vi "Get next JSON Value.vi"() -> (1 "Offset past match":i32, 2 "Value start":i32)   [LabVIEW 2013, in "JSON2.lvlib"]
uses:
  JSON2.lvlib
  JSON Value Search.ctl
panel:
  in  "<JSON> Stream 2":string="[\"string\",\"test2\",\"string\",\"t3\",\"string\", \"string\"]"
  out "Time":dbl format="%#_3p"
  in  "index in":i32
  out "Match":string
  out "Enum":T1=enum."Undefined"
  out "Past Match":string
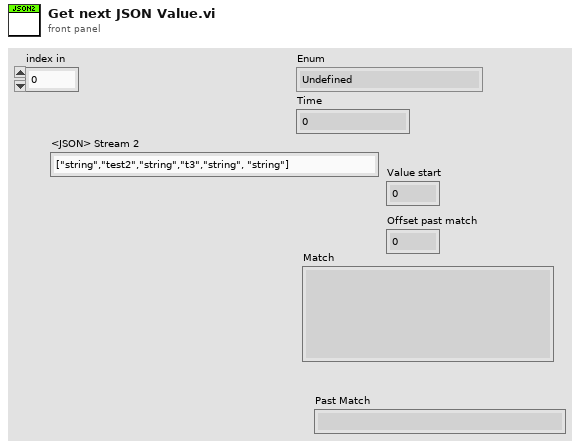
[diagram p1: front panel]
types:
  T1 = typedef "JSON2.lvlib/JSON Value Search.ctl" = enum16{"Parser Error", "In Object", "In Array", "String", "Number", "Leading Whitespace", "Object end", "Array end", "Value end", "Undefined"}
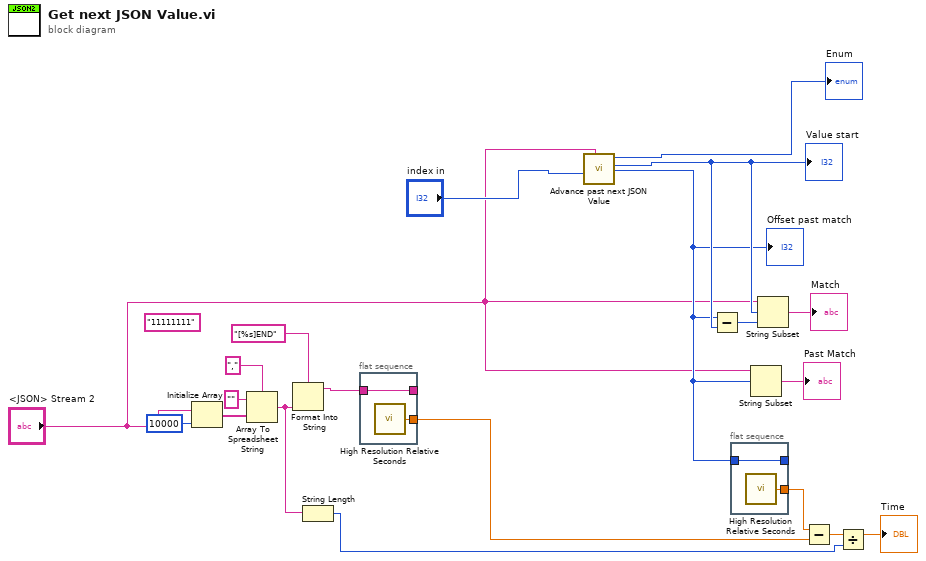
[diagram p0: block diagram]
diagram:
  (unwired) "11111111" ("<JSON> Stream 2")
  n1 = Initialize Array("<JSON> Stream 2", 10000 ("dimension size")) -> (w13:string[])
  n2 = Array To Spreadsheet String(delimiter (Tab)=",", array=w13, 3:"" ("format string")) -> (spreadsheet string=w4:string)
  n3 = Format Into String(format string="[%s]END", w4) -> (resulting string=w9:string)  [unwired: 2 in, 1 out]
  n4 = String Length(string=w4) -> (length=w2:i32)
  n5 = flat-sequence {
    tunnel: [w22] -> _
    tunnel: w9 -> [w22]
    tunnel: [w21] -> w6
    frame #0 {
      n6 = call <vilib>:"High Resolution Relative Seconds.vi"() -> ("relative seconds"=w21:dbl)
    }
  }
  n7 = call "Advance past next JSON Value.vi"("JSON"="<JSON> Stream 2", "Offset"="index in") -> ("index"=w8:i32, "Value start"=w16:i32, "State"=→"Enum":T1)  [unwired: 7 in]
  "Value start" <- w16
  "Offset past match" <- w8
  n8 = Subtract(x=w8, y=w16) -> (x-y=w15:i32)
  n9 = flat-sequence {
    tunnel: [w24] -> _
    tunnel: w8 -> [w24]
    tunnel: [w23] -> w7
    frame #0 {
      n10 = call <vilib>:"High Resolution Relative Seconds.vi"() -> ("relative seconds"=w23:dbl)
    }
  }
  n11 = String Subset(string="<JSON> Stream 2", offset (0)=w8) -> (substring=→"Past Match":string)  [unwired: 1 in]
  n12 = String Subset(string="<JSON> Stream 2", offset (0)=w16, length (rest)=w15) -> (substring=→"Match":string)
  n13 = Subtract(x=w7, y=w6) -> (x-y=w5:dbl)
  n14 = Divide(x=w5, y=w2) -> (x/y=→"Time":dbl)
